vi "Test - Draw Line - Octant 1.vi"() -> ()   [LabVIEW 2022 SP3, in "Raster.lvlib"]
uses:
  Raster.lvlib
  Point 2D (I32).ctl
  Rectangle Dimensions.ctl
  <vilib>/Analysis/baseanly.llb/Mean (DBL).vi
  Utility/Convert Pixels To Picture.vi/d601d993-a776-4dc8-89c7-357d8398c88c.vi
  Utility/Convert Pixels To Picture.vi/7816d0d6-8e4d-41a2-85ac-ed82f1435763.vi
  <vilib>/Utility/High Resolution Relative Seconds.vi
  <vilib>/picture/picture.llb/Draw Unflattened Pixmap.vi
  <vilib>/picture/picture.llb/Draw True-Color Pixmap.vi
  Utility/Utility.lvlib
  <vilib>/Analysis/NI_AALBase.lvlib
panel:
  out "mean":dbl format="%.1p"
  out "new picture":picture
  out "Pixel Data out":u32[][](array[colorbox])
  # "(0,0)"
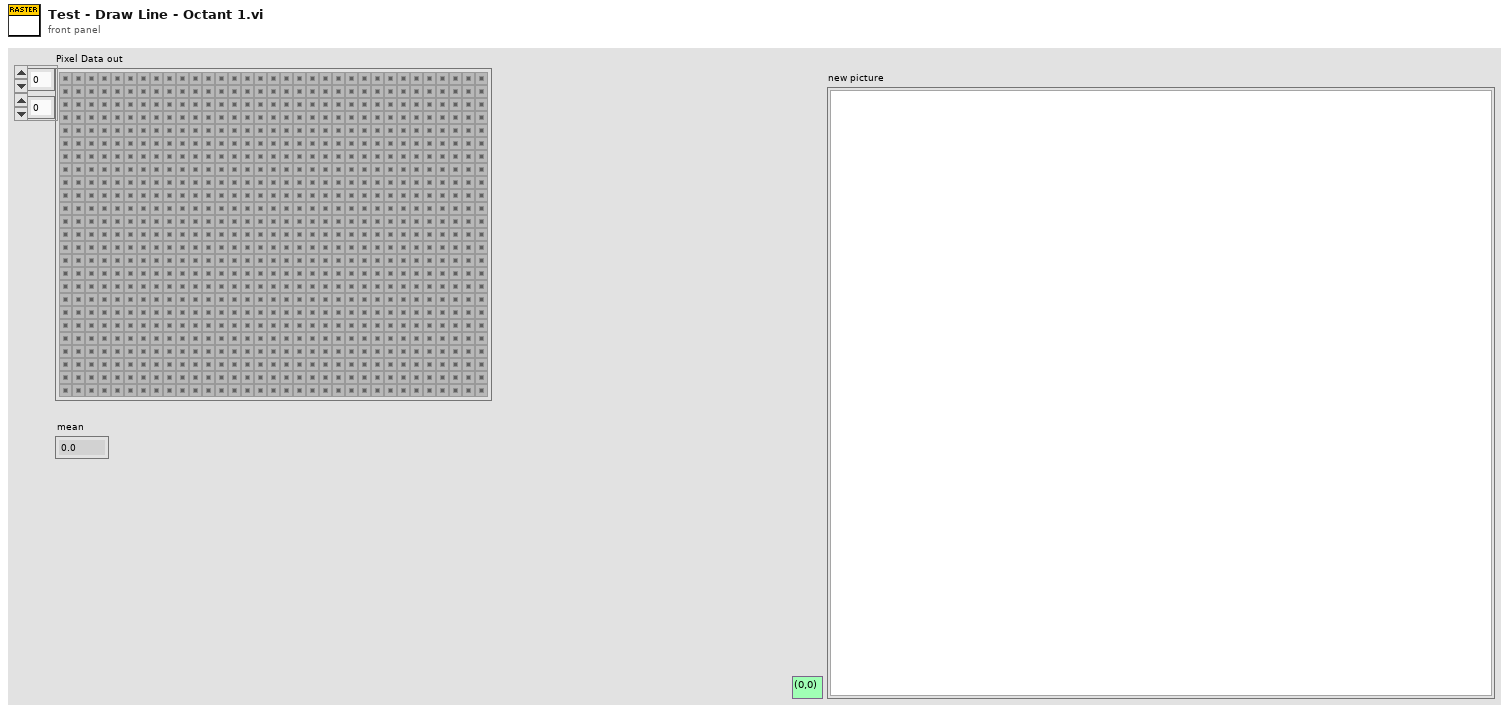
[diagram p1: front panel]
types:
  T1 = typedef "Raster.lvlib/Rectangle Dimensions.ctl" = cluster{"Width":u32, "Height":u32}
  T2 = typedef "Raster.lvlib/Point 2D (I32).ctl" = cluster{"x":i32, "y":i32}
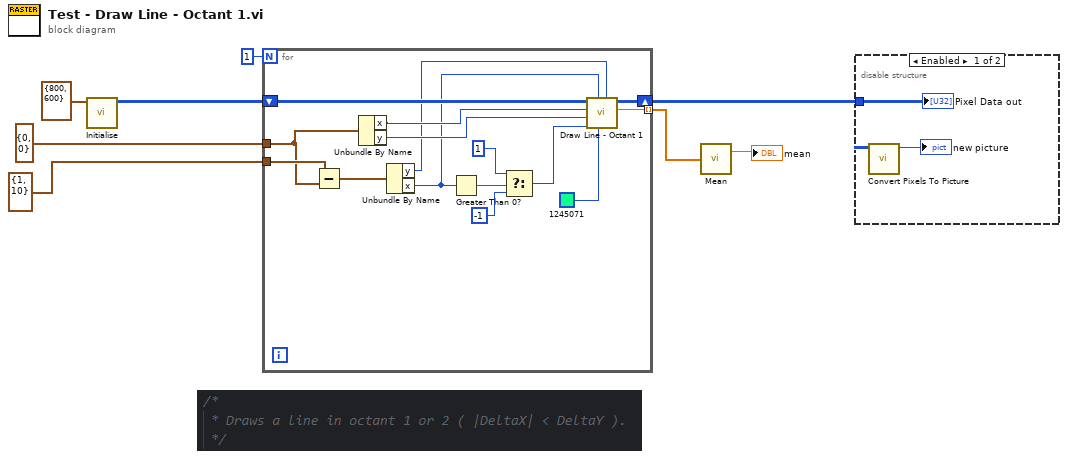
[diagram p0: block diagram]
diagram:
  n1 = call "Initialise.vi"("Screen Dimensions"=T1 {"Width"=800, "Height"=600}) -> ("Pixel Data out"=w7:u32[][])  [unwired: 10 in]
  n2 = for {
    N: 1 -> [_]
    tunnel: [w20] -> w5 mode=indexing
    shift-right: [w22] -> w6
    shift-left: w7 -> [w23]
    tunnel: T2 {"x"=0, "y"=0} ("Point 1") -> [w14]
    tunnel: T2 {"x"=1, "y"=10} ("Point 1") -> [w15]
    n3 = Subtract(x=w15, y=w14) -> (x-y=w18:T2)
    n4 = Unbundle By Name(w14) -> ("x"=w13:i32, "y"=w12:i32)
    n5 = Unbundle By Name(w18) -> ("y"=w10:i32, "x"=w11:i32)
    n6 = Greater Than 0?(x=w11) -> (x > 0?=w19:bool)
    n7 = Select(t=1, s=w19, f=-1 ("t")) -> (s? t:f=w9:i32)
    n8 = call "Draw Line - Octant 1.vi"("Delta y"=w10, "Colour"=u32 1245071, "Delta x"=w11, "x Direction"=w9, "Y0"=w12, "X0"=w13, "Pixel Data in"=w23) -> ("Delta Time [s]"=w20:dbl, "Pixel Data out"=w22:u32[][])  [unwired: 3 in]
  }
  n9 = call-poly <vilib>:"Mean.vi"("X"=w5) -> ("mean"=→"mean":dbl)  [unwired: 1 out]
  n10 = disable-structure shown="Enabled" {
    disable-tunnel: w6 -> [w24 _]
    frame Enabled {
      n11 = call "Convert Pixels To Picture.vi"("Pixel Data in"=w24) -> ("2D Picture"=→"new picture":picture)  [unwired: 9 in, 1 out]
      "Pixel Data out" <- w24
    }
    frame Disabled {
    }
  }
